vi "yokogawa file save pc.vi"() -> ()   [LabVIEW 2011]
panel:
  in  "Unit X":u16(ring) items=["nm", "THz", "cm-1"]
  in  "Unit Y":u16(ring) items=["dBm", "W", "dBm/nm", "W/nm", "W", "dBm/nm", "W/nm"]
  out "Data X Value 2":dbl[](array[numeric]) format="%.4f"
  out "Data Y Value":dbl[](array[numeric]) format="%.4f"
  in  "Select Trace (0: Trace A)":u16(ring) items=["Trace D", "Trace B", "Trace C", "Trace D", "Trace E", "Trace F", "Trace G"]
  out "Error Out":errorcluster
  in  "File Name (USB has to be NTFS format)":string="20150311-#8-fiber-#1"
  in  "Error In":errorcluster
  in  "VISA session":refnum<visa-resource-name>="GPIB0::1::INSTR"
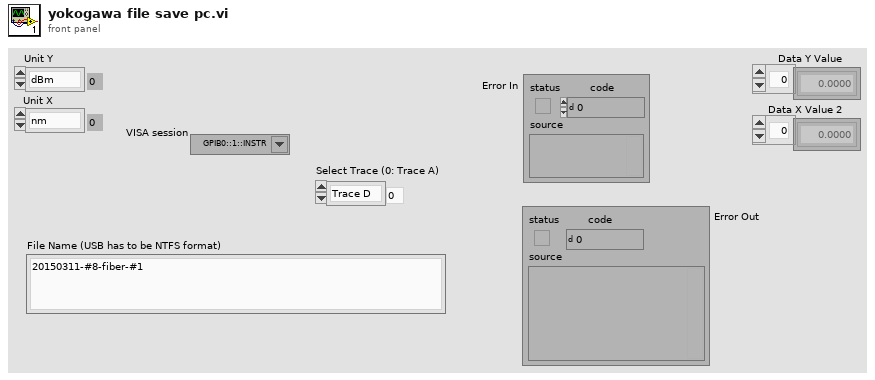
[diagram p1: front panel]
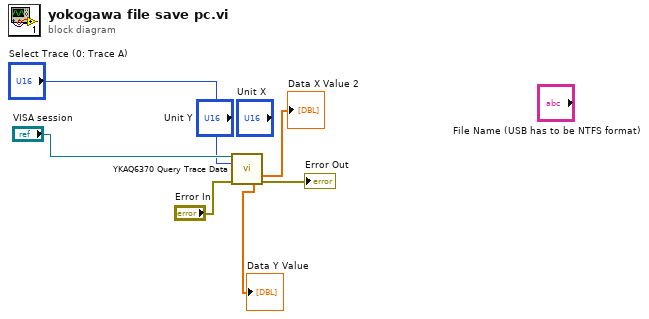
[diagram p0: block diagram]
diagram:
  n1 = call <instrlib>:"YKAQ6370 Query Trace Data.vi"("VISA resource name"="VISA session", "Select Trace  (0: Trace A)"="Select Trace (0: Trace A)", "error in (no error)"="Error In") -> ("Data X Value"=→"Data X Value 2":dbl[], "Data Y Value"=→"Data Y Value":dbl[], "error out"=→"Error Out":errorcluster)  [unwired: 7 in, 3 out]
